vi "SetAd16Default.vi"   [LabVIEW 2014]
uses:
  ESLSCDLL.dll
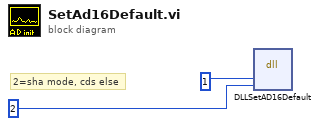
[diagram p0: block diagram]
diagram:
  # "2=sha mode, cds else"
  n1 = dll-call lib="C:/Users/Gerhard/Documents/New64/lv/1cam/board.vis/ESLSCDLL.dll" fn="DLLSetAD16Default"("drv"=u32 1, "res"=u32 2) -> ()  [unwired: 6 in, 2 out]
